vi "Error Handling String.vi"(11 "Auto Err Handling":bool) -> (3 "Error Handling String":string)   [LabVIEW 2023, in "VIDoc Printer.lvlib" / "VIDoc Printer.lvclass"]
doc: "Converts the Auto Error Handling option into a printable String."
uses:
  VIDoc Printer.lvclass
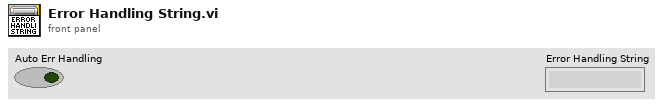
[diagram p1: front panel]
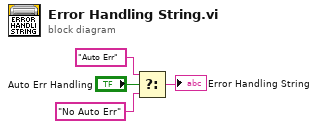
[diagram p0: block diagram]
diagram:
  n1 = Select(t="Auto Err", s="Auto Err Handling", f="No Auto Err") -> (s? t:f=→"Error Handling String":string)
